vi "Parameter_read.vi"(10 "Array":u16[](array[numeric])) -> (3 "Para out":T1)   [LabVIEW 2017]
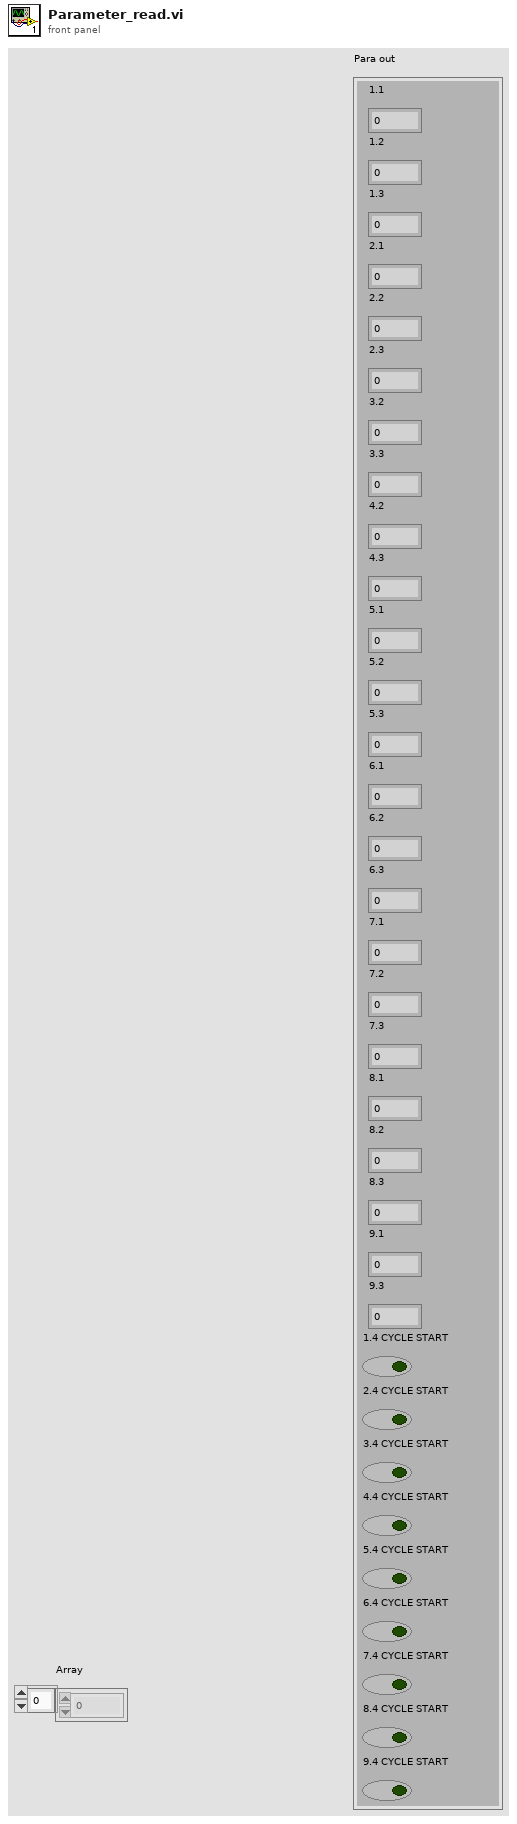
[diagram p1: front panel]
types:
  T1 = cluster{"1.1":dbl, "1.2":dbl, "1.3":dbl, "2.1":dbl, "2.2":dbl, "2.3":dbl, "3.2":dbl, "3.3":dbl, "4.2":dbl, "4.3":dbl, "5.1":dbl, "5.2":dbl, "5.3":dbl, "6.1":dbl, "6.2":dbl, "6.3":dbl, "7.1":dbl, "7.2":dbl, "7.3":dbl, "8.1":dbl, "8.2":dbl, "8.3":dbl, "9.1":dbl, "9.3":dbl, "1.4 CYCLE START":bool, "2.4 CYCLE START":bool, "3.4 CYCLE START":bool, "4.4 CYCLE START":bool, "5.4 CYCLE START":bool, "6.4 CYCLE START":bool, "7.4 CYCLE START":bool, "8.4 CYCLE START":bool, "9.4 CYCLE START":bool}
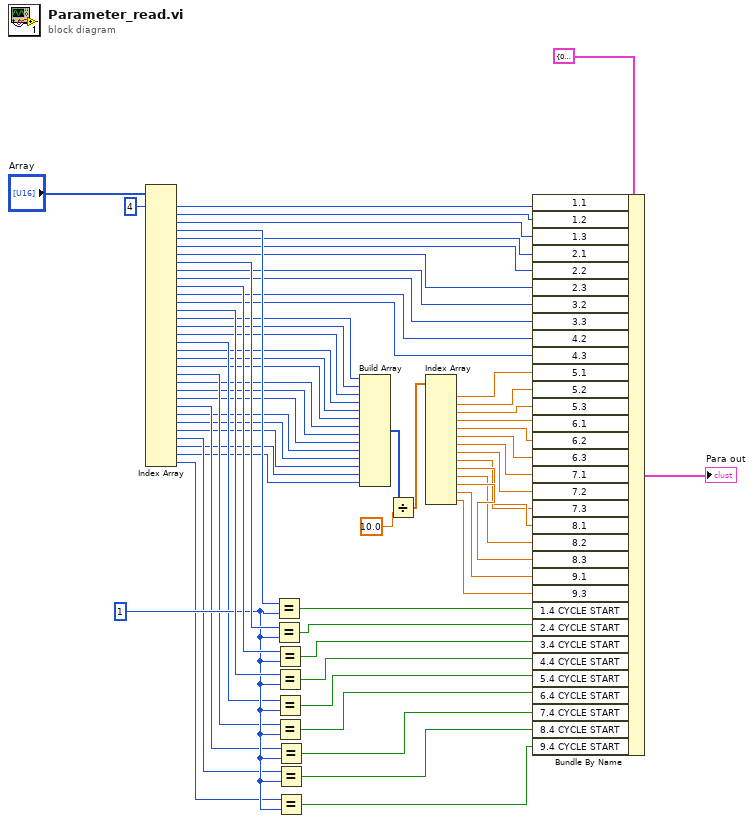
[diagram p0: block diagram]
diagram:
  w43 = 1 ("index")
  n1 = Index Array(array="Array", index #1=4 ("index")) -> (element #1=w62:u16, element #2=w63:u16, element #3=w64:u16, element #4=w59:u16, element #5=w58:u16, element #6=w57:u16, element #7=w56:u16, element #8=w53:u16, element #9=w51:u16, element #10=w50:u16, element #11=w49:u16, element #12=w48:u16, element #13=w47:u16, element #14=w45:u16, element #15=w31:u16, element #16=w30:u16, element #17=w29:u16, element #18=w37:u16, element #19=w28:u16, element #20=w27:u16, element #21=w26:u16, element #22=w36:u16, element #23=w25:u16, element #24=w24:u16, element #25=w23:u16, element #26=w35:u16, element #27=w22:u16, element #28=w21:u16, element #29=w20:u16, element #30=w34:u16, element #31=w19:u16, element #32=w18:u16, element #33=w33:u16)  [unwired: 32 in]
  n2 = Equal?(x=w59, y=w43) -> (x = y?=w54:bool)
  n3 = Equal?(x=w53, y=w43) -> (x = y?=w52:bool)
  n4 = Equal?(x=w49, y=w43) -> (x = y?=w46:bool)
  n5 = Equal?(x=w45, y=w43) -> (x = y?=w44:bool)
  n6 = Equal?(x=w37, y=w43) -> (x = y?=w42:bool)
  n7 = Equal?(x=w36, y=w43) -> (x = y?=w41:bool)
  n8 = Equal?(x=w35, y=w43) -> (x = y?=w40:bool)
  n9 = Equal?(x=w34, y=w43) -> (x = y?=w39:bool)
  n10 = Equal?(x=w33, y=w43) -> (x = y?=w38:bool)
  n11 = Build Array(w31, w30, w29, w28, w27, w26, w25, w24, w23, w22, w21, w20, w19, w18) -> (w17:u16[])
  n12 = Divide(x=w17, y=10.0) -> (x/y=w16:dbl[])
  n13 = Index Array(array=w16) -> (element #1=w2:dbl, element #2=w3:dbl, element #3=w4:dbl, element #4=w5:dbl, element #5=w6:dbl, element #6=w7:dbl, element #7=w8:dbl, element #8=w9:dbl, element #9=w10:dbl, element #10=w11:dbl, element #11=w12:dbl, element #12=w13:dbl, element #13=w14:dbl, element #14=w15:dbl)  [unwired: 14 in]
  n14 = Bundle By Name(cluster=T1 {"1.1"=0.0, "1.2"=0.0, "1.3"=0.0, "2.1"=0.0, "2.2"=0.0, "2.3"=0.0, "3.2"=0.0, "3.3"=0.0, "4.2"=0.0, "4.3"=0.0, "5.1"=0.0, "5.2"=0.0, "5.3"=0.0, "6.1"=0.0, "6.2"=0.0, "6.3"=0.0, "7.1"=0.0, "7.2"=0.0, "7.3"=0.0, "8.1"=0.0, "8.2"=0.0, "8.3"=0.0, "9.1"=0.0, "9.3"=0.0, "1.4 CYCLE START"=FALSE, "2.4 CYCLE START"=FALSE, "3.4 CYCLE START"=FALSE, "4.4 CYCLE START"=FALSE, "5.4 CYCLE START"=FALSE, "6.4 CYCLE START"=FALSE, "7.4 CYCLE START"=FALSE, "8.4 CYCLE START"=FALSE, "9.4 CYCLE START"=FALSE} ("Para out 2"), "1.1"=w62, "1.2"=w63, "1.3"=w64, "2.1"=w58, "2.2"=w57, "2.3"=w56, "3.2"=w51, "3.3"=w50, "4.2"=w48, "4.3"=w47, "5.1"=w2, "5.2"=w3, "5.3"=w4, "6.1"=w5, "6.2"=w6, "6.3"=w7, "7.1"=w8, "7.2"=w9, "7.3"=w10, "8.1"=w11, "8.2"=w12, "8.3"=w13, "9.1"=w14, "9.3"=w15, "1.4 CYCLE START"=w54, "2.4 CYCLE START"=w52, "3.4 CYCLE START"=w46, "4.4 CYCLE START"=w44, "5.4 CYCLE START"=w42, "6.4 CYCLE START"=w41, "7.4 CYCLE START"=w40, "8.4 CYCLE START"=w39, "9.4 CYCLE START"=w38) -> (→"Para out":T1)
